vi "Write Path.vi"(8 "error in (no error)":errorcluster, 9 "Header Description":string, 10 "Path":path, 11 "Logger in":refnum<class "Logger.lvclass">) -> (0 "error out":errorcluster, 3 "Logger out":refnum<class "Logger.lvclass">)   [LabVIEW 2019, in "Logger.lvlib" / "Logger.lvclass"]
uses:
  Logger.lvclass
  Logger.lvclass/Logger.ctl
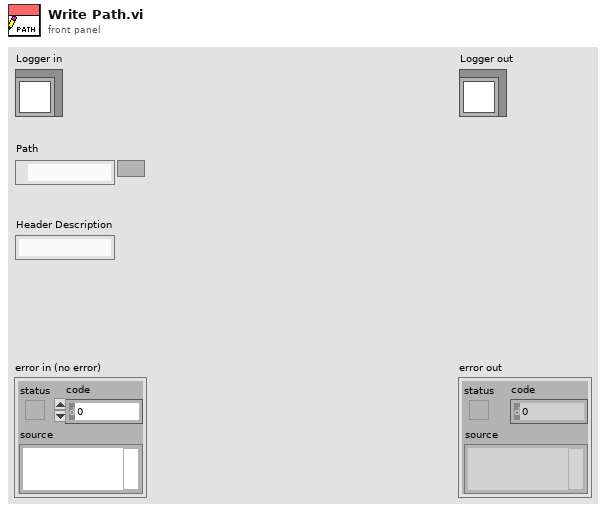
[diagram p1: front panel]
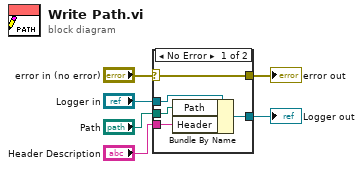
[diagram p0: block diagram]
diagram:
  n1 = case shown="No Error" "error in (no error)" {
    selector: "error in (no error)" -> [w11 w12]
    tunnel: [w11 w12] -> w5
    tunnel: [w9 w13] -> w3
    tunnel: "Logger in" -> [w10 w13]
    tunnel: "Path" -> [w8 _]
    tunnel: "Header Description" -> [w7 _]
    frame No Error {
      n2 = Bundle By Name(cluster=w10, "Path"=w8, "Header"=w7) -> (w9:refnum<class "Logger.lvclass">)
    }
    frame Error {
    }
  }
  "error out" <- w5
  "Logger out" <- w3
